vi "Throw Invalid Name Error.vi"(8 "error in (no error)":errorcluster, 11 "Name":string) -> (0 "error out":errorcluster)   [LabVIEW 2018, in "Instrument Addon Scripting API.lvlib"]
uses:
  Instrument Addon Scripting API.lvlib
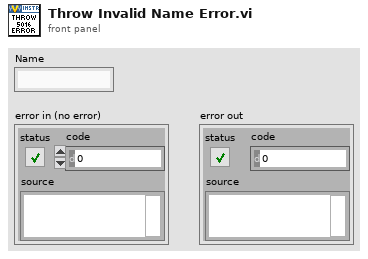
[diagram p1: front panel]
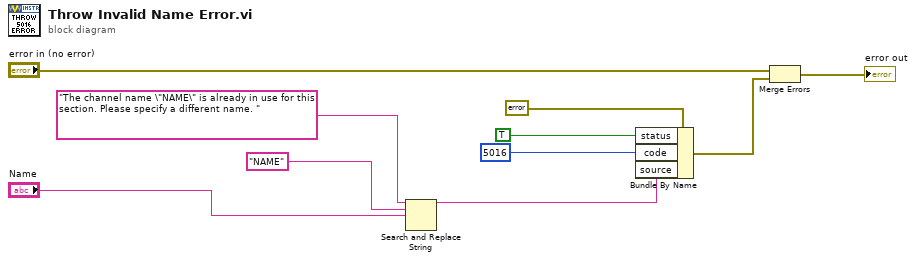
[diagram p0: block diagram]
diagram:
  n1 = Search and Replace String(input string="The channel name \"NAME\" is already in use for this section. Please specify a different name. " ("source"), search string="NAME", replace string="Name") -> (result string=w8:string)  [unwired: 5 in, 3 out]
  n2 = Bundle By Name(cluster=errorcluster {"status"=FALSE, "code"=0, "source"=""} ("error in (no error)"), "status"=TRUE, "code"=5016, "source"=w8) -> (w7:errorcluster)
  n3 = Merge Errors("error in (no error)", w7) -> (→"error out":errorcluster)
